vi "Configure Phase.vi"(8 "error in (no error)":errorcluster, 9 "mode":u8(ring)=1 items=["slave", "master"], 10 "phase, °":dbl, 11 "HFP Gen in":refnum<class "PL HFP Generator.lvclass">) -> (0 "error out":errorcluster, 3 "HFP Gen out":refnum<class "PL HFP Generator.lvclass">)   [LabVIEW 2015, in "PL HFP Generator.lvclass"]
doc: "Configures phase (for Plasma G20 series)."
uses:
  PL HFP Generator.lvclass
  PL HFP Generator.lvclass/PL HFP Generator.ctl
  <vilib>/plasmapper/PL Modbus Client/PL Modbus Client.lvclass
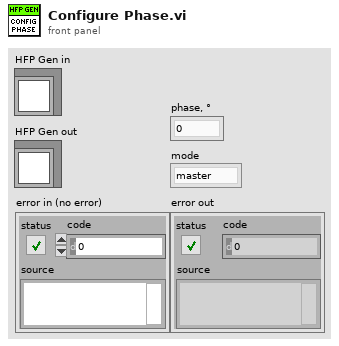
[diagram p1: front panel]
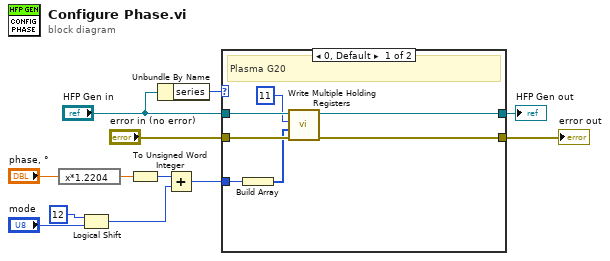
[diagram p0: block diagram]
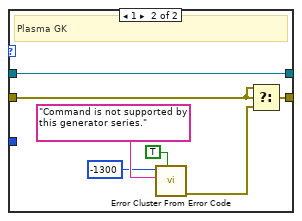
[diagram p2: hidden frame]
diagram:
  n1 = expression code="x*1.2204"("phase, °") -> (w11:dbl)
  n2 = Logical Shift(y=i16 12, x="mode") -> (x << y=w7:u8)
  n3 = To Unsigned Word Integer(number=w11) -> (unsigned 16bit integer=w10:u16)
  n4 = Unbundle By Name("HFP Gen in") -> ("series"=w1:u16)
  n5 = Add(x=w10, y=w7) -> (x+y=w6:u16)
  n6 = case shown="0, Default" w1 {
    tunnel: [w19 w26] -> w5
    tunnel: [w18 w24] -> w4
    tunnel: "error in (no error)" -> [w17 w25]
    tunnel: "HFP Gen in" -> [w16 w26]
    tunnel: w6 -> [w13 _]
    frame 0, Default {
      # "Plasma G20"
      n7 = Build Array(w13) -> (w14:u16[])
      n8 = call <vilib>:"Write Multiple Holding Registers.vi"("error in (no error)"=w17, "values"=w14, "address"=u16 11, "MODBUS in"=w16) -> ("error out"=w18:errorcluster, "MODBUS out"=w19:refnum<class "PL HFP Generator.lvclass">)  [unwired: 6 in]
    }
    frame 1 {
      # "Plasma GK"
      n9 = call <vilib>:"Error Cluster From Error Code.vi"("show call chain? (False)"=TRUE, "error message (\"\")"="Command is not supported by this generator series." ("format string"), "error code (0)"=-1300) -> ("error out"=w20:errorcluster)  [unwired: 6 in]
      n10 = Select(t=w25, s=w25, f=w20) -> (s? t:f=w24:errorcluster)
    }
  }
  "HFP Gen out" <- w5
  "error out" <- w4
